vi "PickTarget.vi"(8 "Find Y? (F)":bool, 10 "Targets Mid":T2(array[cluster]), 11 "Targets Top":T2(array[cluster])) -> (0 "Index":dbl, 1 "Distance (ft)":dbl, 2 "Target Center (-1 to 1)":cluster{"X":dbl, "Y":dbl}, 3 "Chosen Target":T1)   [LabVIEW 2011]
uses:
  Robot Global Data.vi
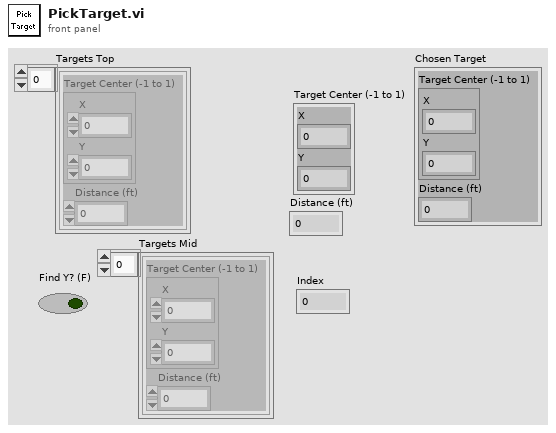
[diagram p1: front panel]
types:
  T1 = cluster{"Target Center (-1 to 1)":cluster{"X":dbl, "Y":dbl}, "Distance (ft)":dbl}
  T2 = cluster{"Target Center (-1 to 1)":cluster{"X":dbl, "Y":dbl}, "Distance (ft)":dbl}[]
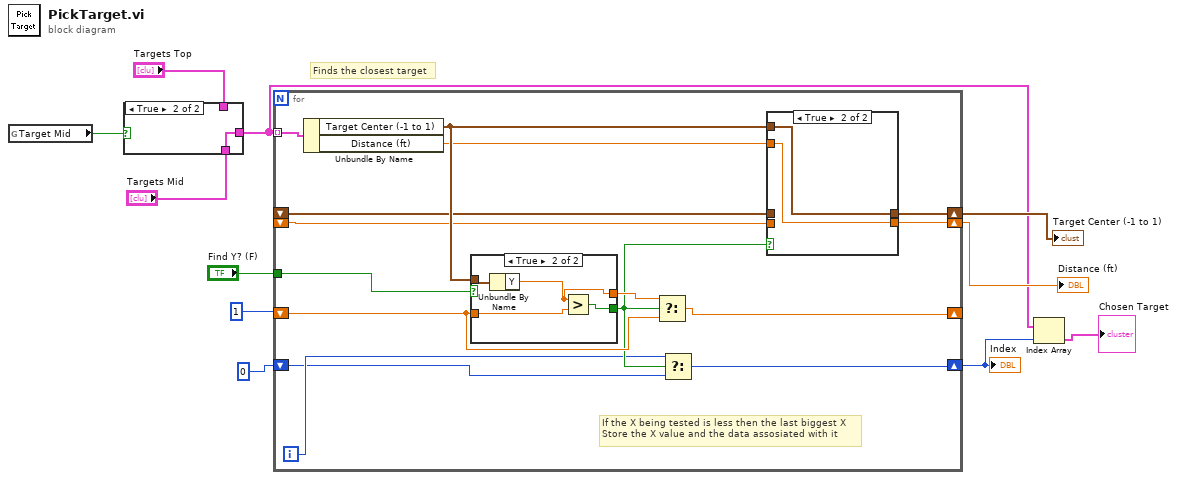
[diagram p0: block diagram]
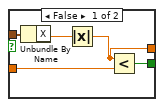
[diagram p3: hidden frame]
diagram:
  # "Finds the closest target"
  n1 = global read "Robot Global Data.vi" "Target Mid"() -> (w6:bool)
  n2 = case shown="True" w6 {
    tunnel: [w12 w13] -> w2
    tunnel: "Targets Top" -> [w12 _]
    tunnel: "Targets Mid" -> [_ w13]
    frame False {
    }
    frame True {
    }
  }
  n3 = for {
    shift-right: [w25] -> w9
    shift-left: _ -> [w23]
    shift-right: [w26] -> w10
    shift-left: _ -> [w24]
    shift-right: [w21] -> _
    shift-left: 1 -> [w22]
    tunnel: "Find Y? (F)" -> [w15]
    shift-right: [w19] -> w3
    shift-left: 0 -> [w16]
    tunnel: w2 -> [w14] mode=indexing
    i -> [w17]
    # "If the X being tested is less then the last biggest X\nStore the X value and the data assosiated with it"
    n4 = Unbundle By Name(w14) -> ("Target Center (-1 to 1)"=w28:cluster{"X":dbl, "Y":dbl}, "Distance (ft)"=w27:dbl)
    n5 = case shown="True" w15 {
      tunnel: w28 -> [w33 w37]
      tunnel: w22 -> [w32 w35]
      tunnel: [w30 w34] -> w20
      tunnel: [w29 w36] -> w18
      frame False {
        n6 = Unbundle By Name(w33) -> ("X"=w31:dbl)
        n7 = Absolute Value(x=w31) -> (abs(x)=w30:dbl)
        n8 = Less?(x=w30, y=w32) -> (x < y?=w29:bool)
      }
      frame True {
        n9 = Unbundle By Name(w37) -> ("Y"=w34:dbl)
        n10 = Greater?(x=w34, y=w35) -> (0:w36:bool)
      }
    }
    n11 = Select(t=w20, s=w18, f=w22) -> (s? t:f=w21:dbl)
    n12 = Select(t=w17, s=w18, f=w16) -> (s? t:f=w19:i32)
    n13 = case shown="True" w18 {
      tunnel: w28 -> [_ w40]
      tunnel: w27 -> [_ w41]
      tunnel: [w38 w41] -> w25
      tunnel: [w39 w40] -> w26
      tunnel: w24 -> [w39 _]
      tunnel: w23 -> [w38 _]
      frame False {
      }
      frame True {
      }
    }
  }
  "Distance (ft)" <- w9
  "Target Center (-1 to 1)" <- w10
  "Index" <- w3
  n14 = Index Array(array=w2, index=w3) -> (element=→"Chosen Target":T1)
